vi "Slider_Module.vi"(7 "Slider":dbl(slide) scale=0.0..10.0, 11 "Error_In":errorcluster) -> (15 "Error_Out":errorcluster)   [LabVIEW 2021]
doc: "This is the main module to generate the data ( Recording the data )"
uses:
  Controls/Operation.ctl
  LV2/UE_C_LV2.vi
  Controls/Event_Data.ctl
  Controls/Event_Data_and_Parameter.ctl
panel:
  out "Record_State":string
  in  "PlayBack?":bool
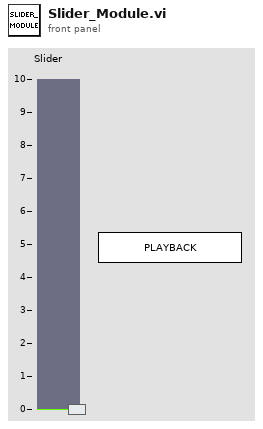
[diagram p1: front panel]
types:
  T1 = typedef "Event_Data.ctl" = cluster{"Event_Data":dbl, "PlayBack?":bool}
  T2 = typedef "Event_Data_and_Parameter.ctl" = cluster{"Event_Data":dbl[], "Generate_Event":bool, "Playback?":bool, "Index":i32}
  T3 = typedef "Operation.ctl" = enum16{"Create_UE", "Generate_UE", "Destroy_UE", "Get_UE_Reference"}
  T4 = enum32{"Bad", "Idle", "Run top level", "Running"}
  T5 = enum16{"Left Button", "Center Button", "Right Button", "Window Close"}
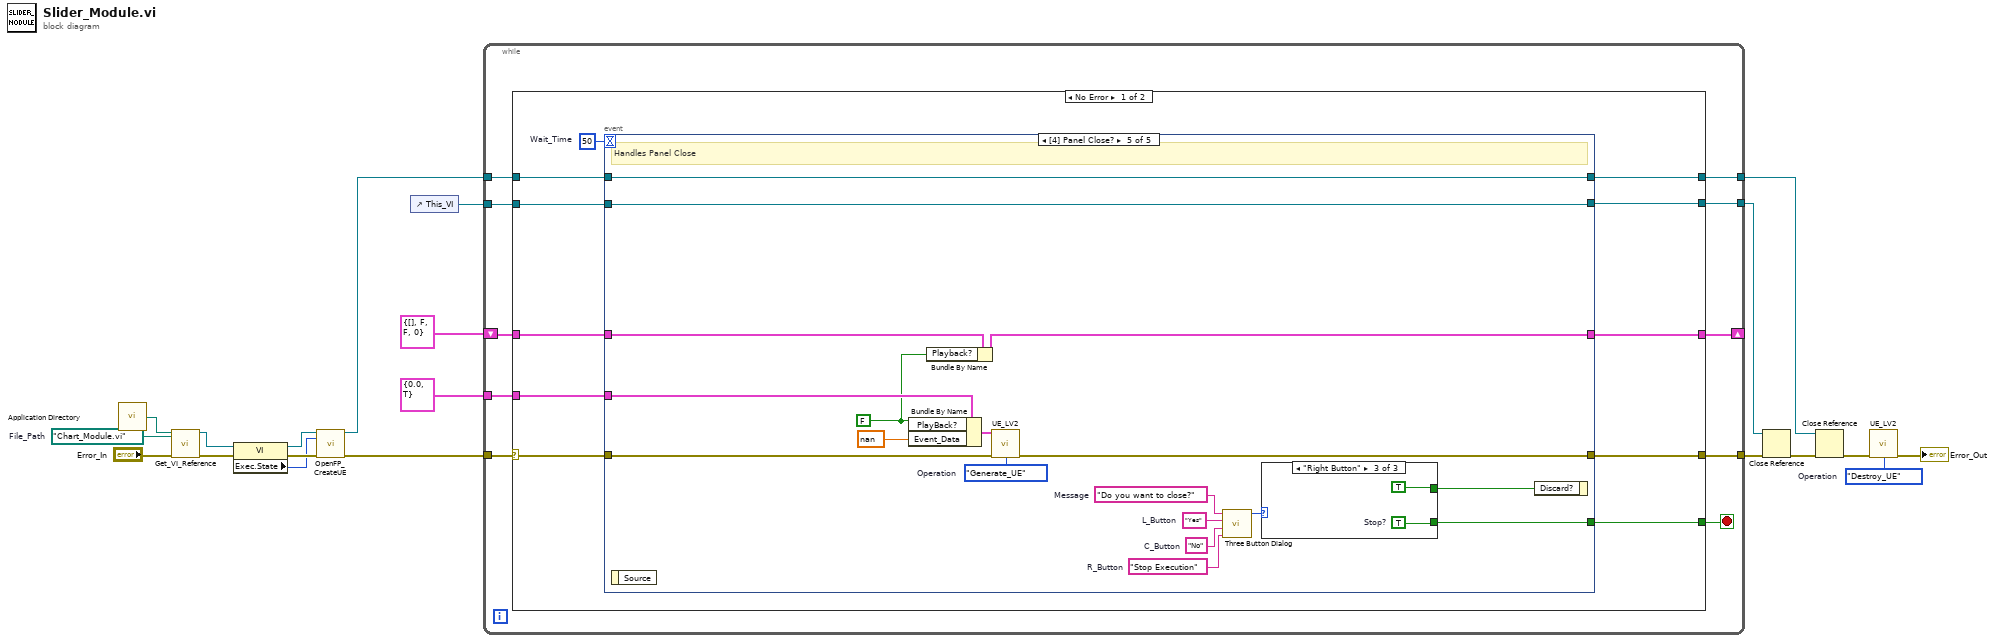
[diagram p0: block diagram]
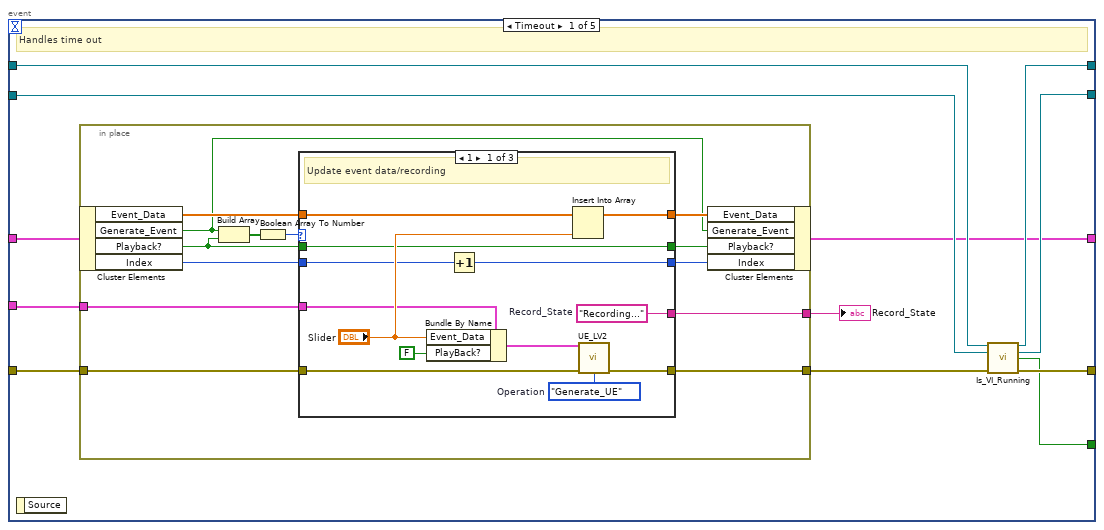
[diagram p2: hidden frame]
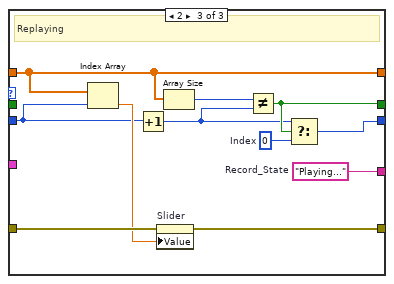
[diagram p4: hidden frame]
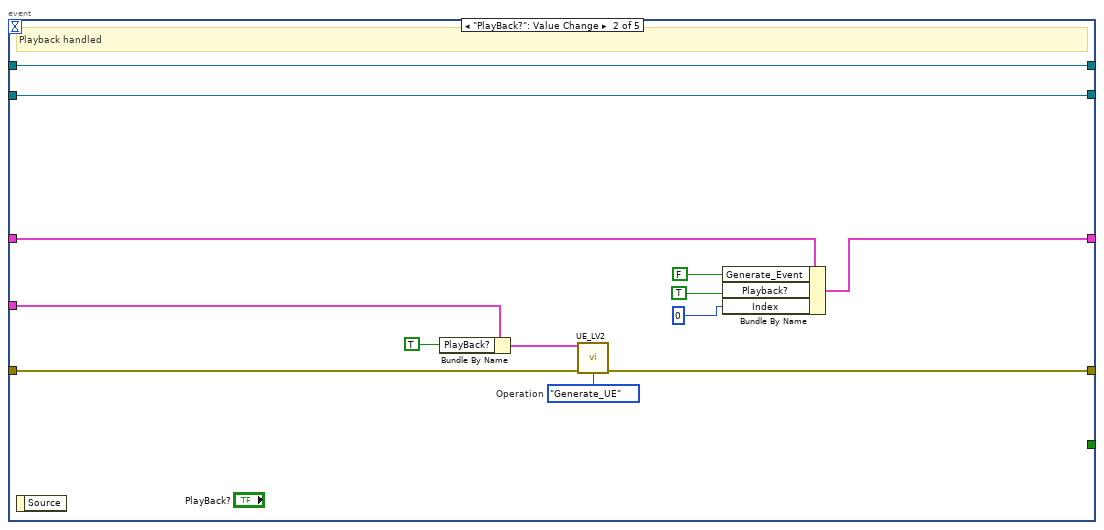
[diagram p5: hidden frame]
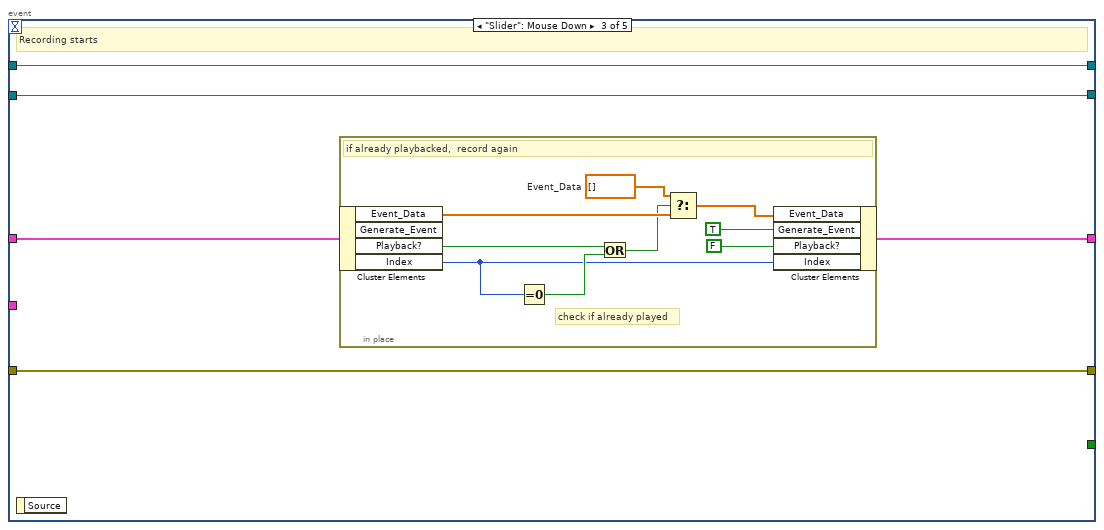
[diagram p6: hidden frame]
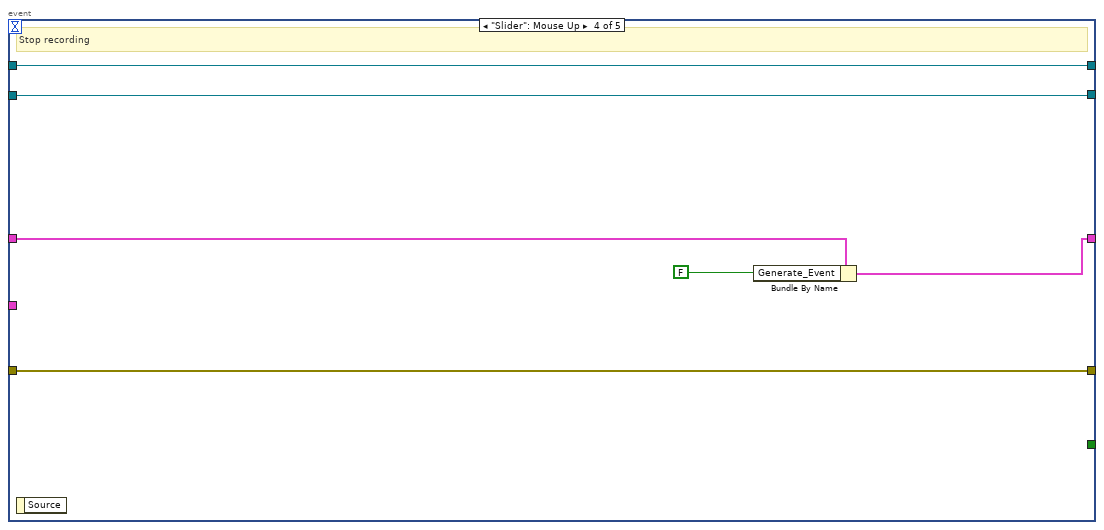
[diagram p7: hidden frame]
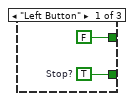
[diagram p8: hidden frame]
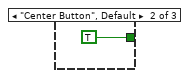
[diagram p9: hidden frame]
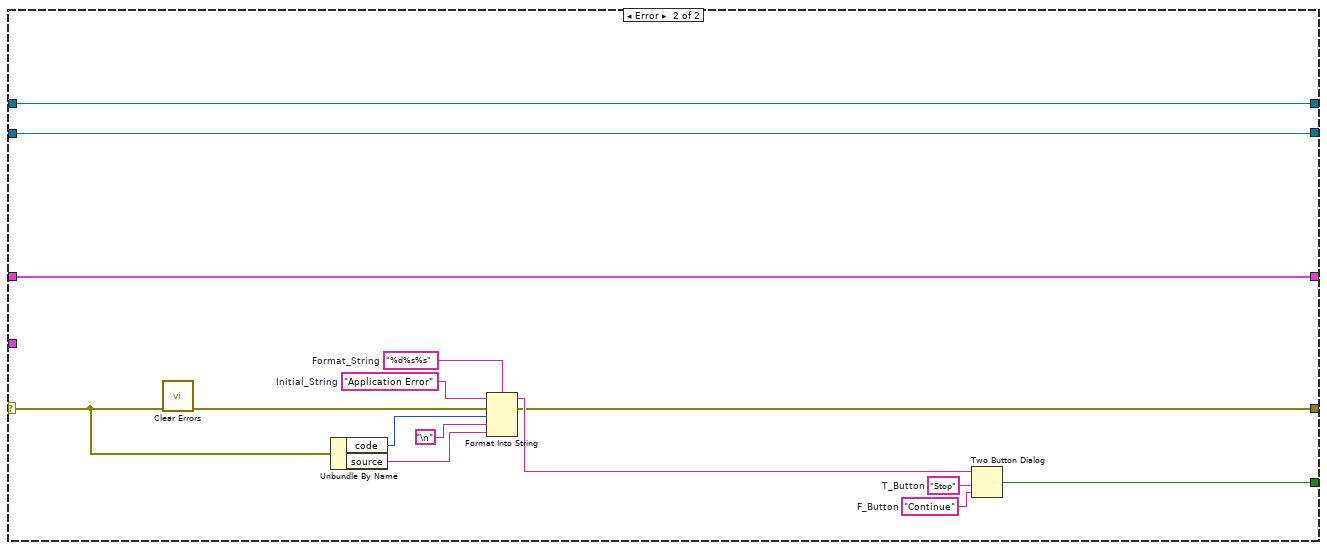
[diagram p10: hidden frame]
diagram:
  w13 = Operation."Destroy_UE"  # Operation
  w17 = path "Chart_Module.vi"  # File_Path
  n1 = call <vilib>:"Application Directory.vi"() -> ("Application Directory"=w18:path)
  n2 = call "Get_VI_Reference.vi"("Application_Directory"=w18, "File_Path"=w17, "Error_In"="Error_In") -> ("VI_Reference"=w16:refnum<vi>, "Error_Out"=w19:errorcluster)  [unwired: 11 in]
  n3 = property on="Property Node" class="VI"(reference=w16, error in=w19) -> (reference out=w5:refnum<vi>, error out=w6:errorcluster, "Exec.State"=w4:T4)
  n4 = call "OpenFP_CreateUE.vi"("VI_Reference_In"=w5, "Exec.State"=w4, "Error_In"=w6) -> ("VI_Reference_Out"=w3:refnum<vi>, "Error_Out"=w2:errorcluster)  [unwired: 11 in]
  n5 = control-ref of="This_VI"() -> (w12:refnum<vi>)
  n6 = while {
    tunnel: w2 -> [w30]
    tunnel: [w29] -> w15
    shift-right: [w27] -> _
    shift-left: T2 {"Event_Data"=[], "Generate_Event"=FALSE, "Playback?"=FALSE, "Index"=0} -> [w26]
    tunnel: w3 -> [w25]
    tunnel: w12 -> [w24]
    tunnel: [w23] -> w11
    tunnel: [w22] -> w8
    tunnel: T1 {"Event_Data"=0.0, "PlayBack?"=TRUE} ("Event_Data") -> [w21]
    stop <- w28 stop-if-true
    n7 = case shown="No Error" w30 {
      selector: w30 -> [w40 w157]
      tunnel: [w41 w158] -> w29
      tunnel: [w38 w154] -> w28
      tunnel: [w32 w153] -> w27
      tunnel: w26 -> [w37 w153]
      tunnel: w25 -> [w36 w152]
      tunnel: w24 -> [w35 w151]
      tunnel: [w34 w151] -> w23
      tunnel: [w33 w152] -> w22
      tunnel: w21 -> [w31 _]
      frame No Error {
        w39 = 50  # Wait_Time
        n8 = event shown="[4] Panel Close?" {
          selector: _ -> [_ _ _ _ _]
          dyn-events: _ -> [_ _ _ _ _]
          timeout: w39 -> [_ _ _ _ _]
          tunnel: [w51 w106 w112 w126 w130] -> w41
          tunnel: w40 -> [w53 w107 w112 w126 w138]
          tunnel: [w46 _ _ _ w131] -> w38
          tunnel: w37 -> [w45 w102 w109 w127 w135]
          tunnel: w36 -> [w50 w96 w111 w123 w139]
          tunnel: w35 -> [w49 w97 w110 w122 w140]
          tunnel: [w48 w97 w110 w122 w140] -> w34
          tunnel: [w47 w96 w111 w123 w139] -> w33
          tunnel: [w44 w101 w108 w125 w134] -> w32
          tunnel: w31 -> [w42 w95 _ _ w133]
          event Timeout {
            # "Handles time out"
            n9 = event-data() -> ()  [unwired: 1 in, 1 out]
            n10 = in-place "In Place Element Structure" {
              in-place-border: w53 -> [w66]
              in-place-border: [w63] -> w52
              in-place-border: [w58] -> w43
              in-place-border: w42 -> [w57]
              n11 = in-place-cluster #1(w45) -> ("Event_Data"=w62:dbl[], "Generate_Event"=w59:bool, "Playback?"=w55:bool, "Index"=w54:i32)
              n12 = Build Array(w59, w55) -> (w65:bool[])
              n13 = Boolean Array To Number(Boolean array=w65) -> (number=w64:u32)
              n14 = case shown="1" w64 {
                tunnel: w66 -> [w79 w81 w94]
                tunnel: [w78 w81 w93] -> w63
                tunnel: [w76 w83 w90] -> w61
                tunnel: w62 -> [w75 w83 w90]
                tunnel: [w67 w82 w88] -> w60
                tunnel: w54 -> [w68 w82 w85]
                tunnel: [w71 _ w91] -> w58
                tunnel: w57 -> [w70 _ _]
                tunnel: [w69 w80 w87] -> w56
                tunnel: w55 -> [w69 w80 _]
                frame 1 {
                  w71 = "Recording..."  # Record_State
                  w77 = Operation."Generate_UE"  # Operation
                  # "Update event data/recording"
                  n15 = Bundle By Name(cluster=w70, "Event_Data"="Slider", "PlayBack?"=FALSE) -> (w73:T1)
                  n16 = Increment(x=w68) -> (x+1=w67:i32)
                  n17 = Insert Into Array(array=w75, new element="Slider") -> (w76:dbl[])  [unwired: 1 in]
                  n18 = call-poly "UE_LV2.vi"("Event_Data"=w73, "Error_In"=w79, "Operation"=w77) -> ("Error_Out"=w78:errorcluster)  [unwired: 11 in, 1 out]
                }
                frame 0, Default {
                  # "No operation"
                }
                frame 2 {
                  w86 = 0  # Index
                  w91 = "Playing..."  # Record_State
                  # "Replaying"
                  n19 = Index Array(array=w90, index=w85) -> (element=w92:dbl)
                  n20 = Increment(x=w85) -> (x+1=w84:i32)
                  n21 = property on="Slider" class="Slide (strict)"(error in=w94, "Value"=w92) -> (error out=w93:errorcluster)  [unwired: 1 in, 1 out]
                  n22 = Array Size(array=w90) -> (size(s)=w89:i32)
                  n23 = Not Equal?(x=w89, y=w84) -> (x != y?=w87:bool)
                  n24 = Select(t=w84, s=w87, f=w86) -> (s? t:f=w88:i32)
                }
              }
              n25 = in-place-cluster #1("Event_Data"=w61, "Generate_Event"=w59, "Playback?"=w56, "Index"=w60) -> (w44:T2)
            }
            "Record_State" <- w43
            n26 = call "Is_VI_Running.vi"("Other_VI_Reference_In"=w50, "This_VI_Reference_In"=w49, "Error_In"=w52) -> ("Other_VI_Reference_Out"=w47:refnum<vi>, "This_VI_Reference_Out"=w48:refnum<vi>, "Stop"=w46:bool, "Error_Out"=w51:errorcluster)  [unwired: 9 in]
          }
          event "PlayBack?": Value Change {
            w105 = Operation."Generate_UE"  # Operation
            # "Playback handled"
            n27 = event-data() -> ()  [unwired: 1 in, 1 out]
            n28 = Bundle By Name(cluster=w95, "PlayBack?"=TRUE) -> (w104:T1)
            n29 = call-poly "UE_LV2.vi"("Event_Data"=w104, "Error_In"=w107, "Operation"=w105) -> ("Error_Out"=w106:errorcluster)  [unwired: 11 in, 1 out]
            n30 = Bundle By Name(cluster=w102, "Generate_Event"=FALSE, "Playback?"=TRUE, "Index"=0) -> (w101:T2)
          }
          event "Slider": Mouse Down {
            # "Recording starts"
            n31 = event-data() -> ()  [unwired: 1 in, 1 out]
            n32 = in-place "In Place Element Structure" {
              w118 = dbl[] []  # Event_Data
              # "check if already played"
              # "if already playbacked,  record again"
              n33 = in-place-cluster #2(w109) -> ("Event_Data"=w117:dbl[], "Playback?"=w113:bool, "Index"=w115:i32)  [unwired: 1 out]
              n34 = Equal To 0?(x=w115) -> (x = 0?=w116:bool)
              n35 = Or(x=w113, y=w116) -> (x .or. y?=w114:bool)
              n36 = Select(t=w118, s=w114, f=w117) -> (s? t:f=w119:dbl[])
              n37 = in-place-cluster #2("Event_Data"=w119, "Generate_Event"=TRUE, "Playback?"=FALSE, "Index"=w115) -> (w108:T2)
            }
          }
          event "Slider": Mouse Up {
            # "Stop recording"
            n38 = event-data() -> ()  [unwired: 1 in, 1 out]
            n39 = Bundle By Name(cluster=w127, "Generate_Event"=FALSE) -> (w125:T2)
          }
          event Panel Close? {
            w128 = FALSE
            w137 = Operation."Generate_UE"  # Operation
            w141 = "Stop Execution"  # R_Button
            w143 = "No"  # C_Button
            w144 = "Yes"  # L_Button
            w145 = "Do you want to close?"  # Message
            # "Handles Panel Close"
            n40 = event-data() -> ()  [unwired: 1 in, 1 out]
            n41 = Bundle By Name(cluster=w133, "PlayBack?"=w128, "Event_Data"=nan) -> (w136:T1)
            n42 = Bundle By Name(cluster=w135, "Playback?"=w128) -> (w134:T2)
            n43 = call-poly "UE_LV2.vi"("Event_Data"=w136, "Error_In"=w138, "Operation"=w137) -> ("Error_Out"=w130:errorcluster)  [unwired: 11 in, 1 out]
            n44 = call <vilib>:"Three Button Dialog.vi"("Right Button Text (\"Cancel\")"=w141, "Center Button Text (\"No\")"=w143, "Left Button Text (\"Yes\")"=w144, "message"=w145) -> ("Which Button?"=w142:T5)  [unwired: 7 in]
            n45 = case shown="\"Right Button\"" w142 {
              tunnel: [FALSE TRUE TRUE] -> w132
              tunnel: [w146 _ w150] -> w131
              frame "Left Button" {
                w146 = TRUE  # Stop?
              }
              frame "Center Button", Default {
              }
              frame "Right Button" {
                w150 = TRUE  # Stop?
              }
            }
            n46 = event-data ("Event Filter Node")("Discard?"=w132) -> ()  [unwired: 1 in, 1 out]
          }
        }
      }
      frame Error {
        w161 = "%d%s%s"  # Format_String
        w162 = "Application Error"  # Initial_String
        w163 = "Stop"  # T_Button
        w164 = "Continue"  # F_Button
        n47 = call <vilib>:"Clear Errors.vi"("error in (no error)"=w157) -> ("error out"=w159:errorcluster)  [unwired: 5 in, 1 out]
        n48 = Unbundle By Name(w157) -> ("code"=w156:i32, "source"=w155:string)
        n49 = Format Into String(format string=w161, initial string=w162, error in=w159, w156, "\n" ("Line Feed Constant"), w155) -> (resulting string=w165:string, error out=w158:errorcluster)
        n50 = Two Button Dialog(message=w165, 1:w164, 2:w163) -> (T button?=w154:bool)
      }
    }
  }
  n51 = Close Reference(reference=w11, error in (no error)=w15) -> (error out=w10:errorcluster)
  n52 = Close Reference(reference=w8, error in (no error)=w10) -> (error out=w9:errorcluster)
  n53 = call-poly "UE_LV2.vi"("Error_In"=w9, "Operation"=w13) -> ("Error_Out"=→"Error_Out":errorcluster)  [unwired: 12 in, 1 out]
